vi "Show_Hide_Controls.vi"(7 "Visible":bool, 10 "error in":errorcluster, 11 "References":T1) -> (2 "error out":errorcluster)   [LabVIEW 2019]
uses:
  TypeDef/#TypeDef_References.ctl
  TypeDef/#TypeDef_Buttons.ctl
  TypeDef/#TypeDef_ReferencesMeassurementProp.ctl
  TypeDef/#TypeDef_ReferencesArchiveProp.ctl
  TypeDef/#TypeDef_Lists.ctl
  TypeDef/#TypeDef_MeasProp.ctl
  TypeDef/#TypeDef_OpProp.ctl
  TypeDef/#TypeDef_Enum_ModeOp.ctl
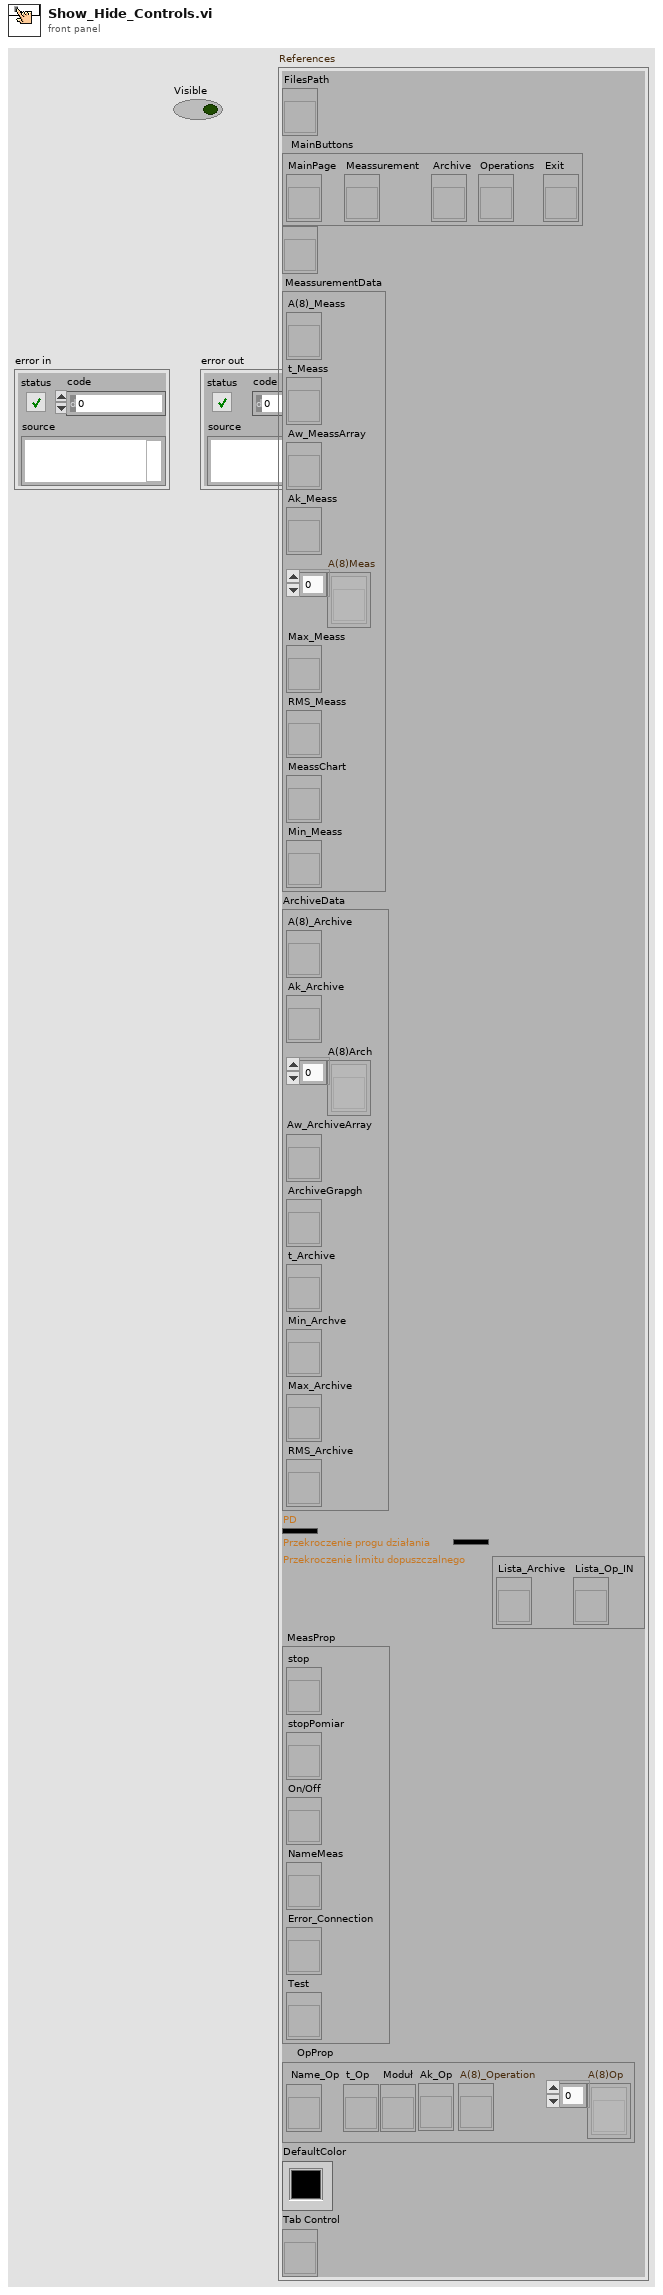
[diagram p1: front panel]
types:
  T1 = typedef "#TypeDef_References.ctl" = cluster{"FilesPath":refnum<vi>, "MainButtons":T2, "Lista CTRL":refnum<vi>, "MeassurementData":T3, "ArchiveData":T4, "PD":u32, "LD":u32, "Lists":T5, "MeasProp":T6, "OpProp":T7, "DefaultColor":u32, "Tab Control":refnum<vi>}
  T2 = typedef "#TypeDef_Buttons.ctl" = cluster{"MainPage":refnum<vi>, "Meassurement":refnum<vi>, "Archive":refnum<vi>, "Operations":refnum<vi>, "Exit":refnum<vi>}
  T3 = typedef "#TypeDef_ReferencesMeassurementProp.ctl" = cluster{"A(8)_Meass":refnum<vi>, "t_Meass":refnum<vi>, "Aw_MeassArray":refnum<vi>, "Ak_Meass":refnum<vi>, "A(8)Meas":refnum<vi>[], "Max_Meass":refnum<vi>, "RMS_Meass":refnum<vi>, "MeassChart":refnum<vi>, "Min_Meass":refnum<vi>}
  T4 = typedef "#TypeDef_ReferencesArchiveProp.ctl" = cluster{"A(8)_Archive":refnum<vi>, "Ak_Archive":refnum<vi>, "A(8)Arch":refnum<vi>[], "Aw_ArchiveArray":refnum<vi>, "ArchiveGrapgh":refnum<vi>, "t_Archive":refnum<vi>, "Min_Archve":refnum<vi>, "Max_Archive":refnum<vi>, "RMS_Archive":refnum<vi>}
  T5 = typedef "#TypeDef_Lists.ctl" = cluster{"Lista_Archive":refnum<vi>, "Lista_Op_IN":refnum<vi>}
  T6 = typedef "#TypeDef_MeasProp.ctl" = cluster{"stop":refnum<vi>, "stopPomiar":refnum<vi>, "On/Off":refnum<vi>, "NameMeas":refnum<vi>, "Error_Connection":refnum<vi>, "Test":refnum<vi>}
  T7 = typedef "#TypeDef_OpProp.ctl" = cluster{"Name_Op":refnum<vi>, "t_Op":refnum<vi>, "Modu³":refnum<vi>, "Ak_Op":refnum<vi>, "A(8)_Operation":refnum<vi>, "A(8)Op":refnum<vi>[]}
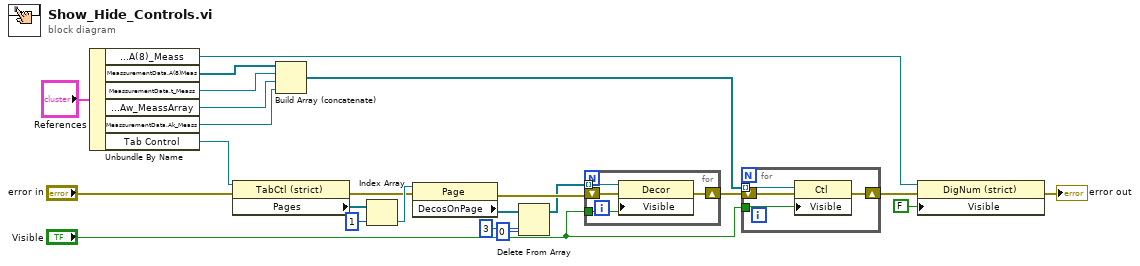
[diagram p0: block diagram]
diagram:
  n1 = Unbundle By Name("References") -> ("MeassurementData.A(8)_Meass"=w16:refnum<vi>, "MeassurementData.A(8)Meas"=w20:refnum<vi>[], "MeassurementData.t_Meass"=w21:refnum<vi>, "MeassurementData.Aw_MeassArray"=w22:refnum<vi>, "MeassurementData.Ak_Meass"=w19:refnum<vi>, "Tab Control"=w13:refnum<vi>)
  n2 = property class="TabCtl (strict)"(reference=w13, error in="error in") -> (error out=w8:errorcluster, "Pages"=w12:refnum<vi>[])  [unwired: 1 out]
  n3 = Build Array (concatenate)(w20, w21, w22, w19) -> (w23:refnum<vi>[])
  n4 = Index Array(array=w12, index=1) -> (element=w11:refnum<vi>)
  n5 = property class="Page"(reference=w11, error in=w8) -> (error out=w9:errorcluster, "DecosOnPage"=w1:refnum<vi>[])  [unwired: 1 out]
  n6 = Delete From Array(array=w1, length=3, index=0) -> (array with subset deleted=w2:refnum<vi>[])  [unwired: 1 out]
  n7 = for {
    tunnel: w2 -> [w25] mode=indexing
    tunnel: "Visible" -> [w24]
    shift-right: [w26] -> w7
    shift-left: w9 -> [w27]
    n8 = property class="Decor"(reference=w25, error in=w27, "Visible"=w24) -> (error out=w26:errorcluster)  [unwired: 1 out]
  }
  n9 = for {
    tunnel: w23 -> [w31] mode=indexing
    shift-right: [w29] -> w18
    shift-left: w7 -> [w30]
    tunnel: "Visible" -> [w28]
    n10 = property class="Ctl"(reference=w31, error in=w30, "Visible"=w28) -> (error out=w29:errorcluster)  [unwired: 1 out]
  }
  n11 = property class="DigNum (strict)"(reference=w16, error in=w18, "Visible"=FALSE) -> (error out=→"error out":errorcluster)  [unwired: 1 out]
